vi "Poll.vi"(8 "error in (no error)":errorcluster, 10 "Switchable Device in":refnum<class "SwitchableDevice.lvclass">, 11 "Button in":refnum<class "Button.lvclass">) -> (0 "error out":errorcluster, 2 "Switchable Device out":refnum<class "SwitchableDevice.lvclass">, 3 "Button out":refnum<class "Button.lvclass">)   [LabVIEW 2018, in "Button.lvclass"]
uses:
  Button.lvclass
  SwitchableDevice_interface/SwitchableDevice.lvclass
  Button.lvclass/Button.ctl
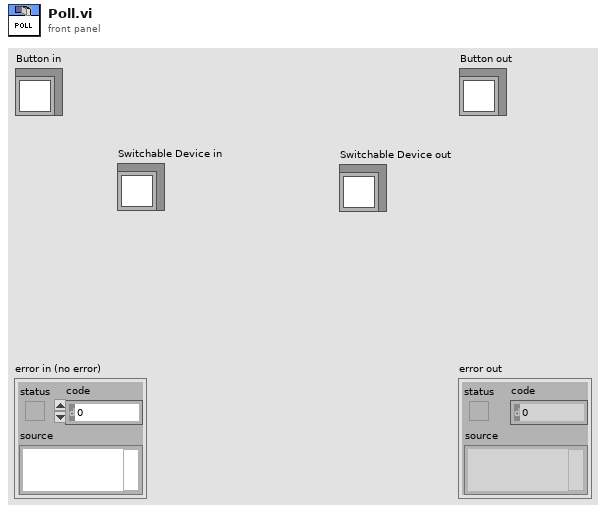
[diagram p1: front panel]
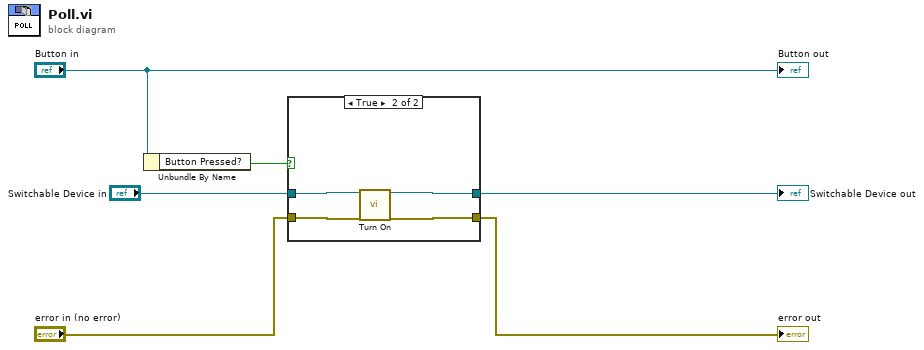
[diagram p0: block diagram]
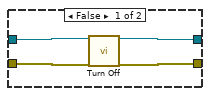
[diagram p2: hidden frame]
diagram:
  n1 = Unbundle By Name("Button in") -> ("Button Pressed?"=w5:bool)
  n2 = case shown="True" w5 {
    tunnel: "Switchable Device in" -> [w10 w13]
    tunnel: "error in (no error)" -> [w9 w14]
    tunnel: [w8 w12] -> w2
    tunnel: [w7 w11] -> w1
    frame False {
      n3 = call "Turn Off.vi"("Interface_object in"=w10, "error in (no error)"=w9) -> ("Interface_object out"=w7:refnum<class "SwitchableDevice.lvclass">, "error out"=w8:errorcluster)  [unwired: 16 in]
    }
    frame True {
      n4 = call "Turn On.vi"("Interface_object in"=w13, "error in (no error)"=w14) -> ("Interface_object out"=w11:refnum<class "SwitchableDevice.lvclass">, "error out"=w12:errorcluster)  [unwired: 16 in]
    }
  }
  "error out" <- w2
  "Switchable Device out" <- w1
  "Button out" <- "Button in"
